vi "Class Path to Variant.vi"(5 "App":refnum<vi>, 11 "Class Path":path) -> (2 "error out":errorcluster, 3 "Class Type":variant)   [LabVIEW 2020, in "FlexBlocks.lvlib"]
uses:
  FlexBlocks.lvlib
  <vilib>/Utility/miscctls.llb/LVPointTypeDef.ctl
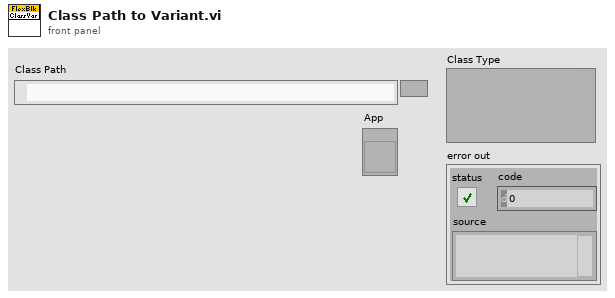
[diagram p1: front panel]
types:
  T1 = typedef "LVPointTypeDef.ctl" = cluster{"Horizontal":i16, "Vertical":i16}
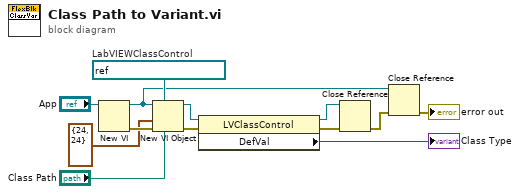
[diagram p0: block diagram]
diagram:
  w12 = refnum<vi> refnum  # LabVIEWClassControl
  n1 = New VI(11:"App") -> (0:w13:errorcluster, 3:w4:refnum<vi>)  [unwired: 6 in]
  n2 = New VI Object(vi object class=w12, owner refnum=w4, position/next to=T1 {"Horizontal"=24, "Vertical"=24} ("location"), 6:"Class Path", 8:w13) -> (object refnum=w11:refnum<vi>, 0:w10:errorcluster)  [unwired: 3 in]
  n3 = property class="LVClassControl"(reference=w11, error in=w10) -> (reference out=w6:refnum<vi>, error out=w7:errorcluster, "DefVal"=→"Class Type":variant)
  n4 = Close Reference(reference=w6, error in (no error)=w7) -> (error out=w5:errorcluster)
  n5 = Close Reference(reference=w4, error in (no error)=w5) -> (error out=→"error out":errorcluster)
